vi "rethinkdb_handshake1.vi"(6 "timeout ms (10000)":i32=10000, 8 "error in (no error)":errorcluster, 10 "version (10=v1_0)":u8=10, 11 "rethinkdb in":refnum<k5>) -> (0 "error out":errorcluster, 2 "server_version":string, 3 "rethinkdb out":refnum<k5>)   [LabVIEW 2017]
uses:
  17f0a6fe-6775-4334-81ae-21231bb255b8.vi
  json/rethinkdb_json_to_cluster.vi
  json/rethinkdb_json_type_cast.vi
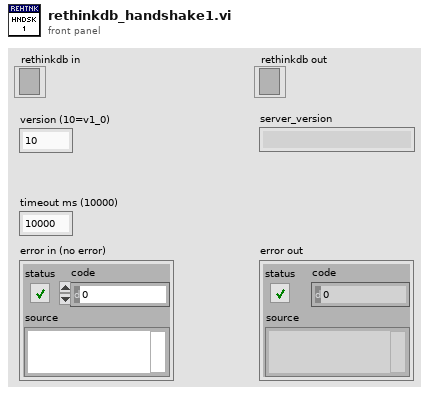
[diagram p1: front panel]
types:
  T1 = cluster{"max_protocol_version":u64, "min_protocol_version":u64, "server_version":string, "success":bool}
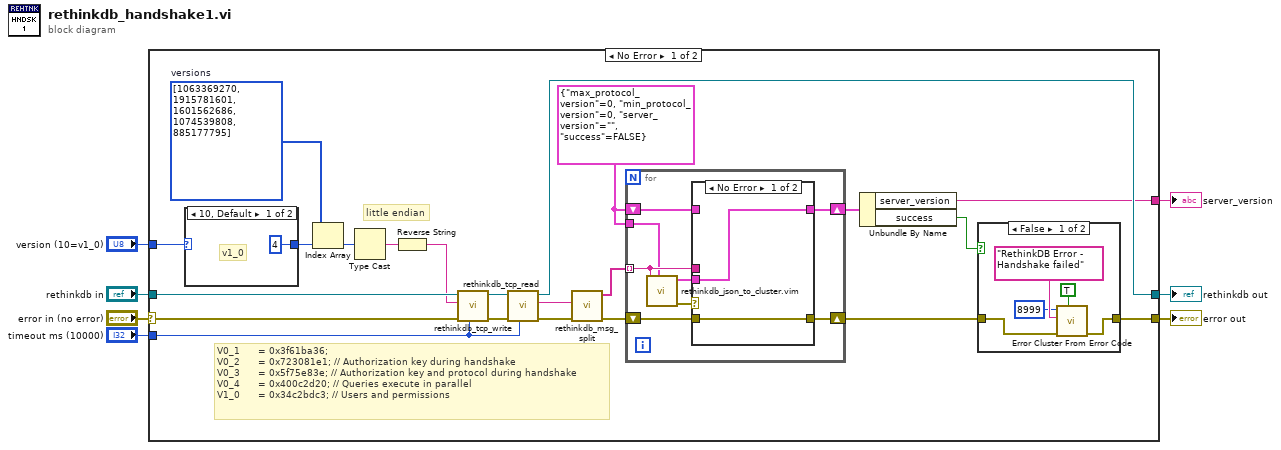
[diagram p0: block diagram]
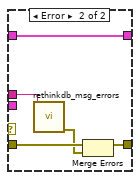
[diagram p2: hidden frame]
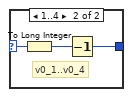
[diagram p3: hidden frame]
diagram:
  n1 = case shown="No Error" "error in (no error)" {
    selector: "error in (no error)" -> [w27 w56]
    tunnel: "version (10=v1_0)" -> [w29 _]
    tunnel: [w12 w56] -> w5
    tunnel: "rethinkdb in" -> [w28 w55]
    tunnel: [w15 w55] -> w3
    tunnel: "timeout ms (10000)" -> [w19 _]
    tunnel: [w8 _] -> w1
    frame No Error {
      w9 = T1 {"max_protocol_version"=0, "min_protocol_version"=0, "server_version"="", "success"=FALSE} ("version")
      w25 = u32[] [1063369270, 1915781601, 1601562686, 1074539808, 885177795]  # versions
      # "little endian"
      # "V0_1      = 0x3f61ba36;\nV0_2      = 0x723081e1; // Authorization key during handshake\nV0_3      = 0x5f75e83e; // Authorization key and protocol during handshake\nV0_4      = 0x400c2d20; // Queries execute in parallel\nV1_0      = 0x34c2bdc3; // Users and permissions"
      n2 = case shown="10, Default" w29 {
        selector: w29 -> [_ w48]
        tunnel: [4 w46] -> w26
        frame 10, Default {
          # "v1_0"
        }
        frame 1..4 {
          # "v0_1..v0_4"
          n3 = To Long Integer(number=w48) -> (32bit integer=w47:i32)
          n4 = Decrement(x=w47) -> (x-1=w46:i32)
        }
      }
      n5 = Index Array(array=w25, index=w26) -> (element=w24:u32)
      n6 = Type Cast(x=w24) -> (*(type *) &x=w23:string)  [unwired: 1 in]
      n7 = Reverse String(1:w23) -> (0:w22:string)
      n8 = call "rethinkdb_tcp_write.vi"("timeout ms (10000)"=w19, "error in (no error)"=w27, "data in"=w22, "rethinkdb in"=w28) -> ("error out"=w21:errorcluster, "rethinkdb out"=w20:refnum<k5>)  [unwired: 5 in, 1 out]
      n9 = call "rethinkdb_tcp_read.vi"("timeout ms (10000)"=w19, "error in (no error)"=w21, "rethinkdb in"=w20) -> ("error out"=w18:errorcluster, "data out"=w14:string, "rethinkdb out"=w15:refnum<k5>)  [unwired: 6 in]
      n10 = call "rethinkdb_msg_split.vi"("error in (no error)"=w18, "data in"=w14) -> ("error out"=w17:errorcluster, "messages"=w16:string[])  [unwired: 7 in, 1 out]
      n11 = for {
        tunnel: w16 -> [w35] mode=indexing
        shift-right: [w34] -> w13
        shift-left: w9 -> [w32]
        tunnel: w9 -> [w31]
        shift-right: [w37] -> w11
        shift-left: w17 -> [w30]
        n12 = call "rethinkdb_json_to_cluster.vim"("type"=w31, "json"=w35) -> ("error out"=w36:errorcluster, "cluster"=w33:T1)  [unwired: 7 in, 1 out]
        n13 = case shown="No Error" w36 {
          tunnel: w35 -> [_ w43]
          tunnel: [w38 w40] -> w37
          tunnel: [w39 w44] -> w34
          tunnel: w33 -> [w39 _]
          tunnel: w32 -> [_ w44]
          tunnel: w30 -> [w38 w42]
          frame No Error {
          }
          frame Error {
            n14 = call "rethinkdb_msg_errors.vi"("message"=w43) -> ("error out"=w41:errorcluster)  [unwired: 10 in]
            n15 = Merge Errors(w42, w41) -> (w40:errorcluster)
          }
        }
      }
      n16 = Unbundle By Name(w13) -> ("server_version"=w8:string, "success"=w10:bool)
      n17 = case shown="False" w10 {
        tunnel: [w49 w54] -> w12
        tunnel: w11 -> [w50 w54]
        frame False {
          n18 = call <vilib>:"Error Cluster From Error Code.vi"("show call chain? (False)"=TRUE, "error in (no error)"=w50, "error message (\"\")"="RethinkDB Error - Handshake failed" ("error message (\"\")"), "error code (0)"=8999) -> ("error out"=w49:errorcluster)  [unwired: 5 in]
        }
        frame True {
        }
      }
    }
    frame Error {
    }
  }
  "error out" <- w5
  "rethinkdb out" <- w3
  "server_version" <- w1
